vi "DFD-DFX_name.vi"() -> (1 "DFD-DFX name":string)   [LabVIEW 2014]
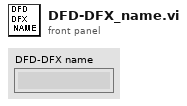
[diagram p1: front panel]
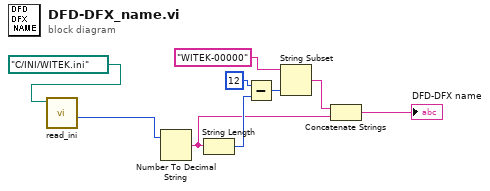
[diagram p0: block diagram]
diagram:
  n1 = call "read_ini.vi"("Path_bench"=path "C:/INI/WITEK.ini") -> ("value"=w4:i64)  [unwired: 10 in]
  n2 = Number To Decimal String(number=w4) -> (decimal integer string=w3:string)  [unwired: 1 in]
  n3 = String Length(string=w3) -> (length=w7:i32)
  n4 = Subtract(x=12, y=w7) -> (x-y=w6:i32)
  n5 = String Subset(string="WITEK-00000", length (rest)=w6) -> (substring=w5:string)  [unwired: 1 in]
  n6 = Concatenate Strings(w5, w3) -> (→"DFD-DFX name":string)
